vi "health_readCfgFile.vi"(8 "error in \n(no error)":errorcluster) -> (0 "error out":errorcluster, 2 "parameters":string[][](array[string]))   [LabVIEW 2018]
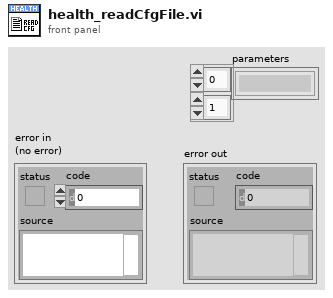
[diagram p1: front panel]
types:
  T1 = enum32{"invalid app kind", "Development System", "Run Time System", "Student Edition", "Embedded LabVIEW", "Evaluation", "Custom"}
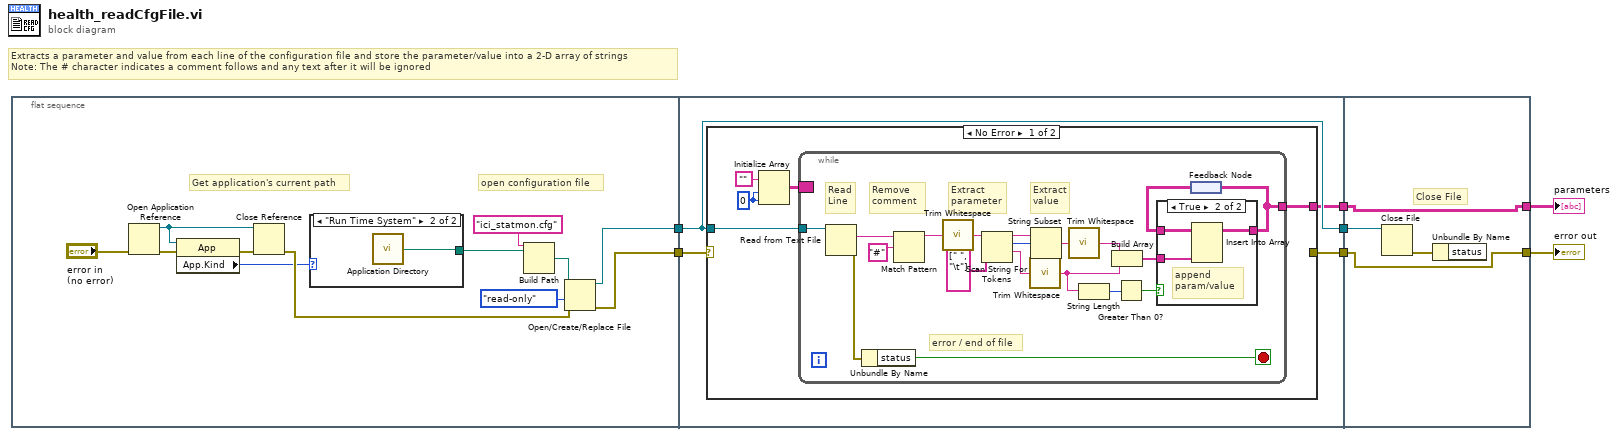
[diagram p0: block diagram]
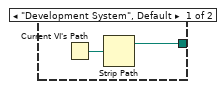
[diagram p2: hidden frame]
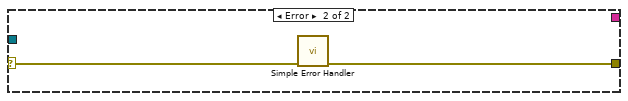
[diagram p4: hidden frame]
diagram:
  # "Extracts a parameter and value from each line of the configuration file and store the parameter/value into a 2-D array of strings\nNote: The # character indicates a comment follows and any text after it will be ignored"
  n1 = flat-sequence {
    tunnel: [w11] -> w5
    tunnel: [w10] -> w4
    tunnel: [w24] -> w3
    tunnel: [w23] -> w2
    tunnel: w5 -> [w26]
    tunnel: [w26] -> w1
    tunnel: w4 -> [w25]
    tunnel: [w58] -> w7
    tunnel: w3 -> [w58]
    tunnel: [w57] -> w6
    tunnel: w2 -> [w57]
    tunnel: w1 -> [w60]
    frame #0 {
      # "open configuration file"
      # "Get application's current path"
      n2 = Open Application Reference(8:"error in \n(no error)") -> (0:w14:errorcluster, 3:w12:refnum<vi>)  [unwired: 3 out]
      n3 = property class="App"(reference=w12, error in=w14) -> (error out=w17:errorcluster, "App.Kind"=w13:T1)  [unwired: 1 out]
      n4 = Close Reference(reference=w12, error in (no error)=w17) -> (error out=w18:errorcluster)
      n5 = case shown="\"Run Time System\"" w13 {
        tunnel: [w20 w22] -> w19
        frame "Development System", Default {
          n6 = Current VI's Path() -> (path=w21:path)
          n7 = Strip Path(path=w21) -> (stripped path=w20:path)  [unwired: 1 out]
        }
        frame "Run Time System" {
          n8 = call <vilib>:"Application Directory.vi"() -> ("Application Directory"=w22:path)
        }
      }
      n9 = Build Path(base path=w19, name or relative path="ici_statmon.cfg") -> (appended path=w16:path)
      n10 = Open/Create/Replace File(file path (use dialog)=w16, error in=w18, access (0:read/write)=enum16{"read/write", "read-only", "write-only"}."read-only") -> (refnum out=w11:refnum<file>, error out=w10:errorcluster)  [unwired: 4 out]
    }
    frame #1 {
      n11 = case shown="No Error" w25 {
        selector: w25 -> [_ w56]
        tunnel: w26 -> [w28 _]
        tunnel: [w27 _] -> w23
        tunnel: [_ w55] -> w24
        frame No Error {
          w29 = 0 ("dimension size")
          n12 = Initialize Array("", w29, w29) -> (w31:string[][])
          n13 = while {
            tunnel: w28 -> [w50]
            border: w31 -> [_]
            tunnel: [w32] -> w27
            stop <- w34 stop-if-true
            # "Read\nLine"
            # "error / end of file"
            # "Remove\ncomment"
            # "Extract\nvalue"
            # "Extract\nparameter"
            n14 = Read from Text File(file (use dialog)=w50) -> (text=w36:string, error out=w48:errorcluster)  [unwired: 1 in, 4 out]
            n15 = Unbundle By Name(w48) -> ("status"=w34:bool)
            n16 = Match Pattern(string=w36, regular expression="#") -> (before substring=w40:string)  [unwired: 4 out]
            n17 = call <vilib>:"Trim Whitespace.vi"("string"=w40) -> ("trimmed string"=w41:string)  [unwired: 1 in]
            n18 = Scan String For Tokens(6:string[] [" ", "\t"] ("delimiters (\\s,\\t,\\r,\\n)"), 9:w41) -> (1:w45:string, 2:w43:i32, 3:w44:string)  [unwired: 1 in, 4 out]
            n19 = call <vilib>:"Trim Whitespace.vi"("string"=w45) -> ("trimmed string"=w37:string)  [unwired: 1 in]
            n20 = String Subset(string=w44, offset (0)=w43) -> (substring=w46:string)  [unwired: 1 in]
            n21 = call <vilib>:"Trim Whitespace.vi"("string"=w46) -> ("trimmed string"=w38:string)  [unwired: 1 in]
            n22 = String Length(string=w37) -> (length=w47:i32)
            n23 = Build Array(w37, w38) -> (w35:string[])
            n24 = Greater Than 0?(x=w47) -> (x > 0?=w33:bool)
            n25 = feedback #1() -> (w49:string[][])
            n26 = case shown="True" w33 {
              tunnel: w49 -> [w51 w54]
              tunnel: [w51 w53] -> w32
              tunnel: w35 -> [_ w52]
              frame False {
              }
              frame True {
                # "append\nparam/value"
                n27 = Insert Into Array(array=w54, new element=w52) -> (w53:string[][])  [unwired: 2 in]
              }
            }
            n28 = feedback-in #1(w32) -> ()
          }
        }
        frame Error {
          n29 = call <vilib>:"Simple Error Handler.vi"("error in (no error)"=w56) -> ("error out"=w55:errorcluster)  [unwired: 4 in, 4 out]
        }
      }
    }
    frame #2 {
      # "Close File"
      n30 = Close File(refnum=w60) -> (error out=w59:errorcluster)  [unwired: 1 in, 1 out]
      n31 = Unbundle By Name(w59) -> ()  [unwired: 1 out]
    }
  }
  "error out" <- w7
  "parameters" <- w6
